vi "Begin.vi"() -> (0 "error out":errorcluster)   [LabVIEW 2011]
doc: "Called before other user functions, this VI is expected to open initial I/O refnums, load in file data, and do all program initialization. Notice that the <B>error out</B> terminal is simply used for data flow. Wiring it to other structures or subVIs ensures that this VI runs first."
uses:
  <vilib>/Rock Robotics/WPI/Camera/WPI_CameraWhite Balance Values.ctl
  <vilib>/Rock Robotics/WPI/Camera/WPI_CameraExposure Values.ctl
  <vilib>/Rock Robotics/WPI/Camera/WPI_CameraFrameRate.ctl
  <vilib>/Rock Robotics/SystemInterfaces/DIO/FPGA_DIOPWMChannel.ctl
  <vilib>/Rock Robotics/WPI/Joystick/WPI_JoystickDeviceEnum.ctl
  <vilib>/Rock Robotics/WPI/MotorControl/WPI_MotorControlOpen Victor.vi
  <vilib>/Rock Robotics/WPI/MotorControl/WPI_MotorControlOpen Jaguar.vi
  Robot Global Data.vi
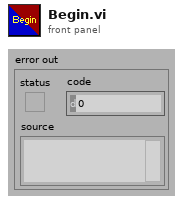
[diagram p1: front panel]
types:
  T1 = typedef "WPI_JoystickDeviceEnum.ctl" = enum16{"USB 1", "USB 2", "USB 3", "USB 4", "Kinect 1", "Kinect 2"}
  T2 = typedef "FPGA_DIOPWMChannel.ctl" = enum8{"PWM 1", "PWM 2", "PWM 3", "PWM 4", "PWM 5", "PWM 6", "PWM 7", "PWM 8", "PWM 9", "PWM 10", "Invalid"}
  T3 = typedef "WPI_CameraFrameRate.ctl" = u32
  T4 = typedef "WPI_CameraExposure Values.ctl" = enum16{"Auto", "Flicker-free 50 Hz", "Flicker-free 60 Hz", "Hold current"}
  T5 = typedef "WPI_CameraWhite Balance Values.ctl" = enum16{"Auto", "Fixed indoor", "Fixed outdoor 1", "Fixed outdoor 2", "Fixed fluorescent 1", "Fixed fluorescent 2", "Hold current"}
  T6 = typedef "WPI_CameraImageSize.ctl" = enum16{"640x480", "320x240", "160x120"}
  T7 = typedef "WPI_CameraDevRef.ctl" = cluster{"Camera Address":string, "CameraStatus":errorcluster, "Acquire Image Notifier":refnum<notifier>}
  T8 = typedef "WPI_ServoDeviceRef.ctl" = cluster{"DeviceStatus":errorcluster, "Digital Module":T9, "PWM Channel":T2, "DeadBand":T10}
  T9 = typedef "FPGA_TypedefDigitalModule.ctl" = enum16{"Digital Module 1", "Digital Module 2"}
  T10 = typedef "WPI_PWMDeadband.ctl" = cluster{"Name":string, "maxPositivePwm":i32, "minPositivePwm":i32, "centerPwm":i32, "maxNegativePwm":i32, "minNegativePwm":i32, "angularRange":u16}
  T11 = typedef "WPI_MotorControlDeviceRef.ctl" = cluster{"DeviceStatus":errorcluster, "Type":enum16{"PWM", "CAN"}, "PWM":cluster{"Digital Module":T9, "PWM Channel":T2, "DeadBand":T10}, "CAN":cluster{"Device Number":u8, "Control Mode":T12, "Semaphore":T13, "Max Vout":dbl}, "Invert":bool, "TransformRef":T14, "InvTransformRef":T14}
  T12 = typedef "WPI_CANJaguar_ControlMode.ctl" = enum8{"Percent VBus", "Current", "Speed", "Position", "Voltage"}
  T13 = typedef "Semaphore RefNum" = refnum<k1>
  T14 = typedef "WPI_PWMTransform_ConPane.ctl" = refnum<vi>
  T15 = typedef "WPI_JoystickDevRef.ctl" = cluster{"Device":T1}
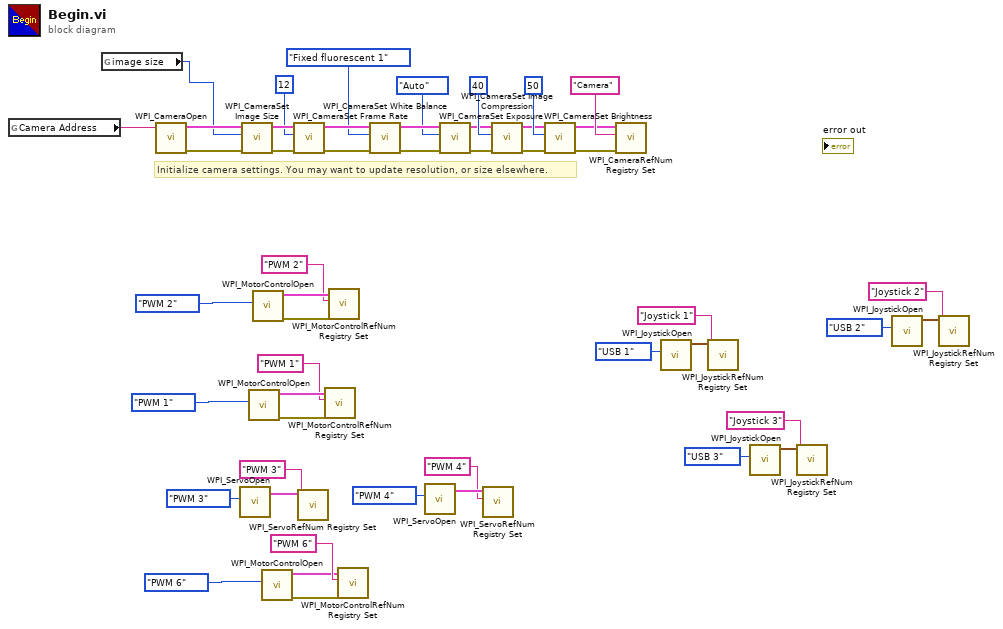
[diagram p0: block diagram]
diagram:
  # "Initialize camera settings. You may want to update resolution, or size elsewhere."
  n1 = global read "Robot Global Data.vi" "Camera Address"() -> (w29:string)
  n2 = global read "Robot Global Data.vi" "image size"() -> (w28:T6)
  n3 = call <vilib>:"WPI_CameraOpen.vi"("Camera Address"=w29) -> ("error out"=w40:errorcluster, "CameraDevRef"=w41:T7)  [unwired: 1 in, 8 out]
  n4 = call <vilib>:"WPI_ServoOpen.vi"("PWM Channel"=FPGA_DIOPWMChannel."PWM 3") -> ("ServoDeviceRef"=w14:T8)  [unwired: 9 in, 1 out]
  n5 = call <vilib>:"WPI_CameraSet Image Size.vi"("error in (no error)"=w40, "Image Size"=w28, "CameraDevRef"=w41) -> ("error out"=w39:errorcluster, "CameraDevRef Out"=w42:T7)  [unwired: 7 out]
  n6 = call-poly <vilib>:"WPI_MotorControlOpen.vi"("PWM Channel"=FPGA_DIOPWMChannel."PWM 1") -> ("error out"=w20:errorcluster, "MotorControlDeviceRef"=w23:T11)  [unwired: 9 in]
  n7 = call-poly <vilib>:"WPI_MotorControlOpen.vi"("PWM Channel"=FPGA_DIOPWMChannel."PWM 2") -> ("error out"=w21:errorcluster, "MotorControlDeviceRef"=w26:T11)  [unwired: 9 in]
  n8 = call-poly <vilib>:"WPI_MotorControlOpen.vi"("PWM Channel"=FPGA_DIOPWMChannel."PWM 6") -> ("error out"=w9:errorcluster, "MotorControlDeviceRef"=w7:T11)  [unwired: 9 in]
  n9 = call <vilib>:"WPI_CameraSet Frame Rate.vi"("error in (no error)"=w39, "Frame Rate (fps)"=T3 12, "CameraDevRef"=w42) -> ("error out"=w38:errorcluster, "CameraDevRef Out"=w44:T7)  [unwired: 7 out]
  n10 = call <vilib>:"WPI_ServoRefNum Registry Set.vi"("refnum name"="PWM 3", "ServoDeviceRef"=w14) -> ()  [unwired: 8 in, 2 out]
  n11 = call <vilib>:"WPI_MotorControlRefNum Registry Set.vi"("error in (no error)"=w20, "refnum name"="PWM 1", "MotorControlDevRef"=w23) -> ()  [unwired: 7 in, 2 out]
  n12 = call <vilib>:"WPI_MotorControlRefNum Registry Set.vi"("error in (no error)"=w21, "refnum name"="PWM 2", "MotorControlDevRef"=w26) -> ()  [unwired: 7 in, 2 out]
  n13 = call <vilib>:"WPI_MotorControlRefNum Registry Set.vi"("error in (no error)"=w9, "refnum name"="PWM 6", "MotorControlDevRef"=w7) -> ()  [unwired: 7 in, 2 out]
  n14 = call <vilib>:"WPI_CameraSet White Balance.vi"("error in (no error)"=w38, "White Balance"=WPI_CameraWhite_Balance_Values."Fixed fluorescent 1", "CameraDevRef"=w44) -> ("error out"=w37:errorcluster, "CameraDevRef Out"=w43:T7)  [unwired: 7 out]
  n15 = call <vilib>:"WPI_ServoOpen.vi"("PWM Channel"=FPGA_DIOPWMChannel."PWM 4") -> ("ServoDeviceRef"=w12:T8)  [unwired: 9 in, 1 out]
  n16 = call <vilib>:"WPI_CameraSet Exposure.vi"("error in (no error)"=w37, "Exposure"=WPI_CameraExposure_Values."Auto", "CameraDevRef"=w43) -> ("error out"=w36:errorcluster, "CameraDevRef Out"=w46:T7)  [unwired: 7 out]
  n17 = call <vilib>:"WPI_ServoRefNum Registry Set.vi"("refnum name"="PWM 4", "ServoDeviceRef"=w12) -> ()  [unwired: 8 in, 2 out]
  n18 = call <vilib>:"WPI_CameraSet Image Compression.vi"("error in (no error)"=w36, "Compression"=40, "CameraDevRef"=w46) -> ("error out"=w35:errorcluster, "CameraDevRef Out"=w45:T7)  [unwired: 7 out]
  n19 = call <vilib>:"WPI_CameraSet Brightness.vi"("error in (no error)"=w35, "Brightness"=50, "CameraDevRef"=w45) -> ("error out"=w33:errorcluster, "CameraDevRef Out"=w34:T7)  [unwired: 7 out]
  n20 = call <vilib>:"WPI_CameraRefNum Registry Set.vi"("error in (no error)"=w33, "refnum name"="Camera", "CameraDevRef"=w34) -> ()  [unwired: 9 out]
  n21 = call <vilib>:"WPI_JoystickOpen.vi"("JoystickDevice"=WPI_JoystickDeviceEnum."USB 1") -> ("JoystickDevRef"=w19:T15)  [unwired: 10 in]
  n22 = call <vilib>:"WPI_JoystickRefNum Registry Set.vi"("refnum name"="Joystick 1", "JoystickDevRef"=w19) -> ()  [unwired: 8 in, 2 out]
  n23 = call <vilib>:"WPI_JoystickOpen.vi"("JoystickDevice"=WPI_JoystickDeviceEnum."USB 3") -> ("JoystickDevRef"=w4:T15)  [unwired: 10 in]
  n24 = call <vilib>:"WPI_JoystickRefNum Registry Set.vi"("refnum name"="Joystick 3", "JoystickDevRef"=w4) -> ()  [unwired: 8 in, 2 out]
  n25 = call <vilib>:"WPI_JoystickOpen.vi"("JoystickDevice"=WPI_JoystickDeviceEnum."USB 2") -> ("JoystickDevRef"=w16:T15)  [unwired: 10 in]
  n26 = call <vilib>:"WPI_JoystickRefNum Registry Set.vi"("refnum name"="Joystick 2", "JoystickDevRef"=w16) -> ()  [unwired: 8 in, 2 out]
